vi "test_RS-xxx Read.vi"(8 "error in (no error)":errorcluster, 11 "TestCase in":refnum<class "Instrument Addon Serial Protocols Unit Tests.lvclass">) -> (0 "error out":errorcluster, 3 "TestCase out":refnum<class "Instrument Addon Serial Protocols Unit Tests.lvclass">)   [LabVIEW 2023, in "Instrument Addon Serial Protocols Unit Tests.lvclass"]
uses:
  Instrument Addon Serial Protocols Unit Tests.lvclass
  Instrument Addon Serial Protocols Unit Tests.lvclass/Instrument Addon Serial Protocols Unit Tests.ctl
  <vilib>/addons/_JKI Toolkits/VI Tester/TestCase.llb/TestCase.lvclass
  Listener/Listener.lvclass
  Listener/ListenerClassControls/Operation.ctl
  <vilib>/platform/TimedLoop/XDataNode/XDataNode.xnode
  <vilib>/Platform/TimedLoop/XDataNode/nitl_modes.ctl
  <vilib>/Platform/TimedLoop/XDataNode/XDNodeRunTimeDep.lvlib
  <vilib>/Platform/TimedLoop/XDataNode/wakeup.ctl
  <vilib>/Platform/TimedLoop/XDataNode/timing_clust.ctl
  RS-xxx/RS-xxx.lvclass
  Protocol Parent/Methods/Read Parameter.ctl
  Protocol Parent/Protocol Parent.lvclass
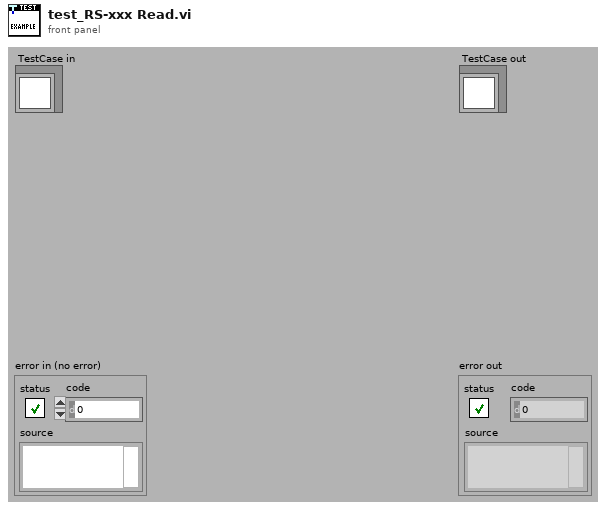
[diagram p1: front panel]
types:
  T1 = typedef "Protocols.lvlib/Protocol Parent.lvclass/Read Parameter.ctl" = cluster{"Wait Type":enum16{"Byte Count", "Wait sec"}, "Wait Value":dbl}
  T2 = typedef "Listener.lvclass/Operation.ctl" = enum16{"Read", "Write"}
  T3 = typedef "XDNodeRunTimeDep.lvlib/timing_clust.ctl" = cluster{"Expected End [f-1]":u64, "Actual End [f-1]":u64, "Finished Late? [f-1]":bool, "Expected End [i-1]":u64, "Actual End [i-1]":u64, "Finished Late? [i-1]":bool, "Expected Start [i]":u64, "Actual Start [i]":u64, "Expected Start [f]":u64, "Actual Start [f]":u64, "Source Name":string, "Structure Name":string, "Period":i64, "Deadline":i64, "Offset":i64, "Start":i64, "Priority":i32, "Timeout":i32, "Mode":T4, "Wakeup Reason":T5, "Error":errorcluster, "Source Type":string, "Secondary Source Type":string, "Global End Time":u64, "Global Start Time":u64, "Frame Duration":u64, "Iteration Duration":u64, "Assigned CPU":i32, "I/O Scan Engine Mode":u32}
  T4 = typedef "XDNodeRunTimeDep.lvlib/nitl_modes.ctl" = enum32{"No Change", "Process missed periods, maintain original phase", "Discard missed periods, maintain original phase", "Process missed periods, ignore original phase", "Discard missed periods, ignore original phase"}
  T5 = typedef "XDNodeRunTimeDep.lvlib/wakeup.ctl" = enum32{"Normal", "Aborted", "Asynchronous wakeup", "Timing source error", "Timed loop error", "Timeout"}
  T6 = typedef "Listener.lvclass/RS-xxx Data Structure.ctl" = cluster{"Virtual COM Port Settings 1":cluster{"Port":string, "Baud Rate":u32, "Data Bits":u16, "Parity":enum16{"None", "Odd", "Even", "Mark", "Space"}, "Stop Bits":u16, "Flow Control":u16, "XON":enum16{"NUL", "SOH", "STX", "ETX", "EOT", "ENQ", "ACK", "BEL", "BS", "HT", "LF", "VT", "FF", "CR", "SO", "SI", "DLE", "DC1", "DC2", "DC3", "DC4", "NAK", "SYN", "ETB", "CAN", "EM", "SUB", "ESC", "FS", "GS", "RS", "US", "SP", "!", "\"", "#", "$", "%", "&", "'", "(", ")", "*", "+", ",", "- (-)", ".", "/", "0", "1", "2", "3", "4", "5", "6", "7", "8", "9", ":", ";", "<", "=", ">", "?", "@", "A", "B", "C", "D", "E", "F", "G", "H", "I", "J", "K", "L", "M", "N", "O", "P", "Q", "R", "S", "T", "U", "V", "W", "X", "Y", "Z", "[", "\\", "]", "^", "_", "`", "a", "b", "c", "d", "e", "f", "g", "h", "i", "j", "k", "l", "m", "n", "o", "p", "q", "r", "s", "t", "u", "v", "w", "x", "y", "z", "{", "|", "}", "~"}, "XOFF":enum16{"NUL", "SOH", "STX", "ETX", "EOT", "ENQ", "ACK", "BEL", "BS", "HT", "LF", "VT", "FF", "CR", "SO", "SI", "DLE", "DC1", "DC2", "DC3", "DC4", "NAK", "SYN", "ETB", "CAN", "EM", "SUB", "ESC", "FS", "GS", "RS", "US", "SP", "!", "\"", "#", "$", "%", "&", "'", "(", ")", "*", "+", ",", "- (-)", ".", "/", "0", "1", "2", "3", "4", "5", "6", "7", "8", "9", ":", ";", "<", "=", ">", "?", "@", "A", "B", "C", "D", "E", "F", "G", "H", "I", "J", "K", "L", "M", "N", "O", "P", "Q", "R", "S", "T", "U", "V", "W", "X", "Y", "Z", "[", "\\", "]", "^", "_", "`", "a", "b", "c", "d", "e", "f", "g", "h", "i", "j", "k", "l", "m", "n", "o", "p", "q", "r", "s", "t", "u", "v", "w", "x", "y", "z", "{", "|", "}", "~"}, "End Read on Termination Character":bool, "End Write on Termination Character":bool, "Termination Character":u8}, "Virtual COM Port Settings 2":cluster{"Port":string, "Baud Rate":u32, "Data Bits":u16, "Parity":enum16{"None", "Odd", "Even", "Mark", "Space"}, "Stop Bits":u16, "Flow Control":u16, "XON":enum16{"NUL", "SOH", "STX", "ETX", "EOT", "ENQ", "ACK", "BEL", "BS", "HT", "LF", "VT", "FF", "CR", "SO", "SI", "DLE", "DC1", "DC2", "DC3", "DC4", "NAK", "SYN", "ETB", "CAN", "EM", "SUB", "ESC", "FS", "GS", "RS", "US", "SP", "!", "\"", "#", "$", "%", "&", "'", "(", ")", "*", "+", ",", "- (-)", ".", "/", "0", "1", "2", "3", "4", "5", "6", "7", "8", "9", ":", ";", "<", "=", ">", "?", "@", "A", "B", "C", "D", "E", "F", "G", "H", "I", "J", "K", "L", "M", "N", "O", "P", "Q", "R", "S", "T", "U", "V", "W", "X", "Y", "Z", "[", "\\", "]", "^", "_", "`", "a", "b", "c", "d", "e", "f", "g", "h", "i", "j", "k", "l", "m", "n", "o", "p", "q", "r", "s", "t", "u", "v", "w", "x", "y", "z", "{", "|", "}", "~"}, "XOFF":enum16{"NUL", "SOH", "STX", "ETX", "EOT", "ENQ", "ACK", "BEL", "BS", "HT", "LF", "VT", "FF", "CR", "SO", "SI", "DLE", "DC1", "DC2", "DC3", "DC4", "NAK", "SYN", "ETB", "CAN", "EM", "SUB", "ESC", "FS", "GS", "RS", "US", "SP", "!", "\"", "#", "$", "%", "&", "'", "(", ")", "*", "+", ",", "- (-)", ".", "/", "0", "1", "2", "3", "4", "5", "6", "7", "8", "9", ":", ";", "<", "=", ">", "?", "@", "A", "B", "C", "D", "E", "F", "G", "H", "I", "J", "K", "L", "M", "N", "O", "P", "Q", "R", "S", "T", "U", "V", "W", "X", "Y", "Z", "[", "\\", "]", "^", "_", "`", "a", "b", "c", "d", "e", "f", "g", "h", "i", "j", "k", "l", "m", "n", "o", "p", "q", "r", "s", "t", "u", "v", "w", "x", "y", "z", "{", "|", "}", "~"}, "End Read on Termination Character":bool, "End Write on Termination Character":bool, "Termination Character":u8}, "Data":string, "Data Length":u32}
  T7 = cluster{"Port":string, "Baud Rate":u32, "Data Bits":u16, "Parity":enum16{"None", "Odd", "Even", "Mark", "Space"}, "Stop Bits":u16, "Flow Control":u16, "XON":enum16{"NUL", "SOH", "STX", "ETX", "EOT", "ENQ", "ACK", "BEL", "BS", "HT", "LF", "VT", "FF", "CR", "SO", "SI", "DLE", "DC1", "DC2", "DC3", "DC4", "NAK", "SYN", "ETB", "CAN", "EM", "SUB", "ESC", "FS", "GS", "RS", "US", "SP", "!", "\"", "#", "$", "%", "&", "'", "(", ")", "*", "+", ",", "- (-)", ".", "/", "0", "1", "2", "3", "4", "5", "6", "7", "8", "9", ":", ";", "<", "=", ">", "?", "@", "A", "B", "C", "D", "E", "F", "G", "H", "I", "J", "K", "L", "M", "N", "O", "P", "Q", "R", "S", "T", "U", "V", "W", "X", "Y", "Z", "[", "\\", "]", "^", "_", "`", "a", "b", "c", "d", "e", "f", "g", "h", "i", "j", "k", "l", "m", "n", "o", "p", "q", "r", "s", "t", "u", "v", "w", "x", "y", "z", "{", "|", "}", "~"}, "XOFF":enum16{"NUL", "SOH", "STX", "ETX", "EOT", "ENQ", "ACK", "BEL", "BS", "HT", "LF", "VT", "FF", "CR", "SO", "SI", "DLE", "DC1", "DC2", "DC3", "DC4", "NAK", "SYN", "ETB", "CAN", "EM", "SUB", "ESC", "FS", "GS", "RS", "US", "SP", "!", "\"", "#", "$", "%", "&", "'", "(", ")", "*", "+", ",", "- (-)", ".", "/", "0", "1", "2", "3", "4", "5", "6", "7", "8", "9", ":", ";", "<", "=", ">", "?", "@", "A", "B", "C", "D", "E", "F", "G", "H", "I", "J", "K", "L", "M", "N", "O", "P", "Q", "R", "S", "T", "U", "V", "W", "X", "Y", "Z", "[", "\\", "]", "^", "_", "`", "a", "b", "c", "d", "e", "f", "g", "h", "i", "j", "k", "l", "m", "n", "o", "p", "q", "r", "s", "t", "u", "v", "w", "x", "y", "z", "{", "|", "}", "~"}, "End Read on Termination Character":bool, "End Write on Termination Character":bool, "Termination Character":u8}
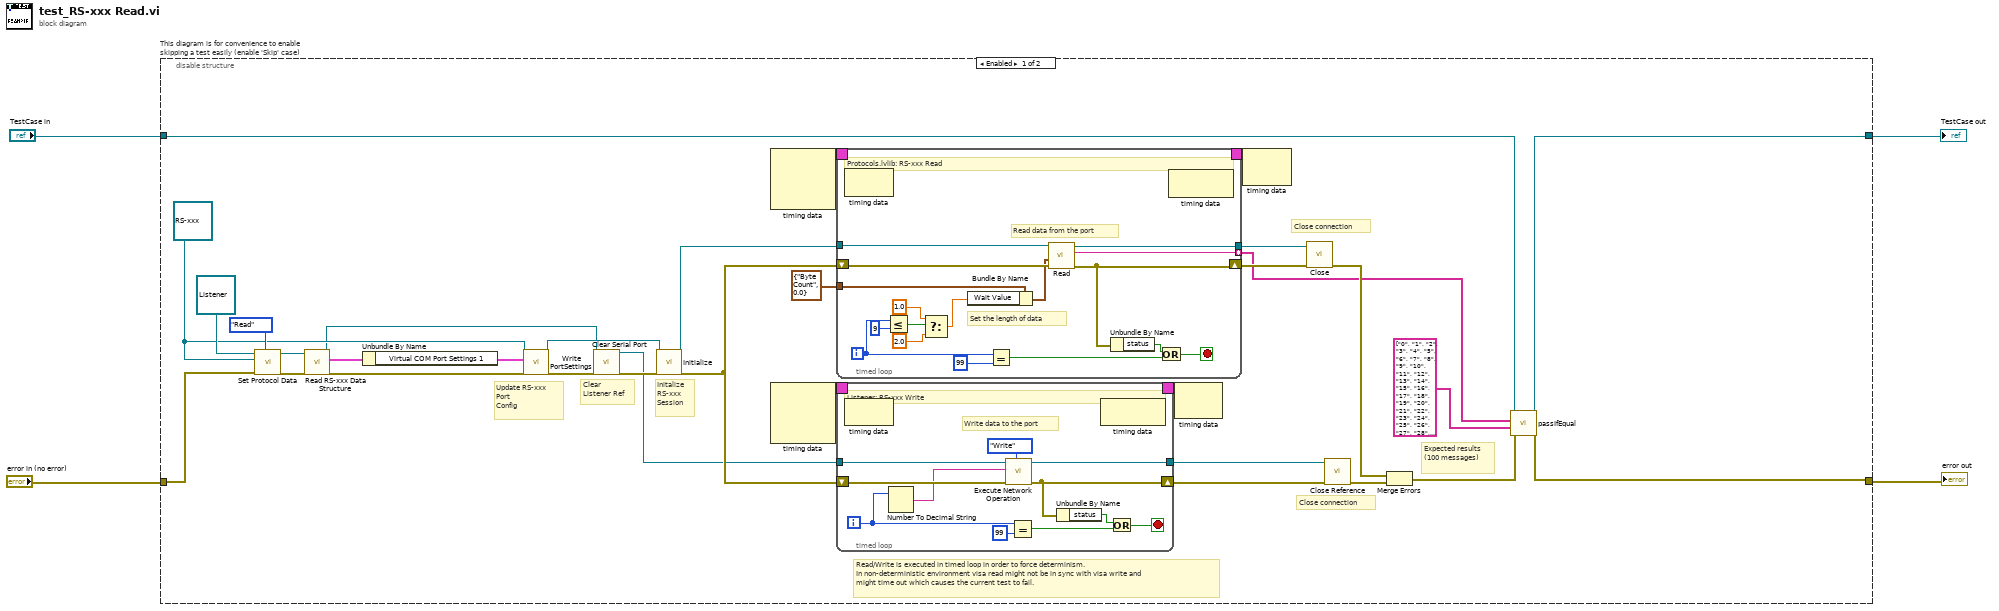
[diagram p0: block diagram]
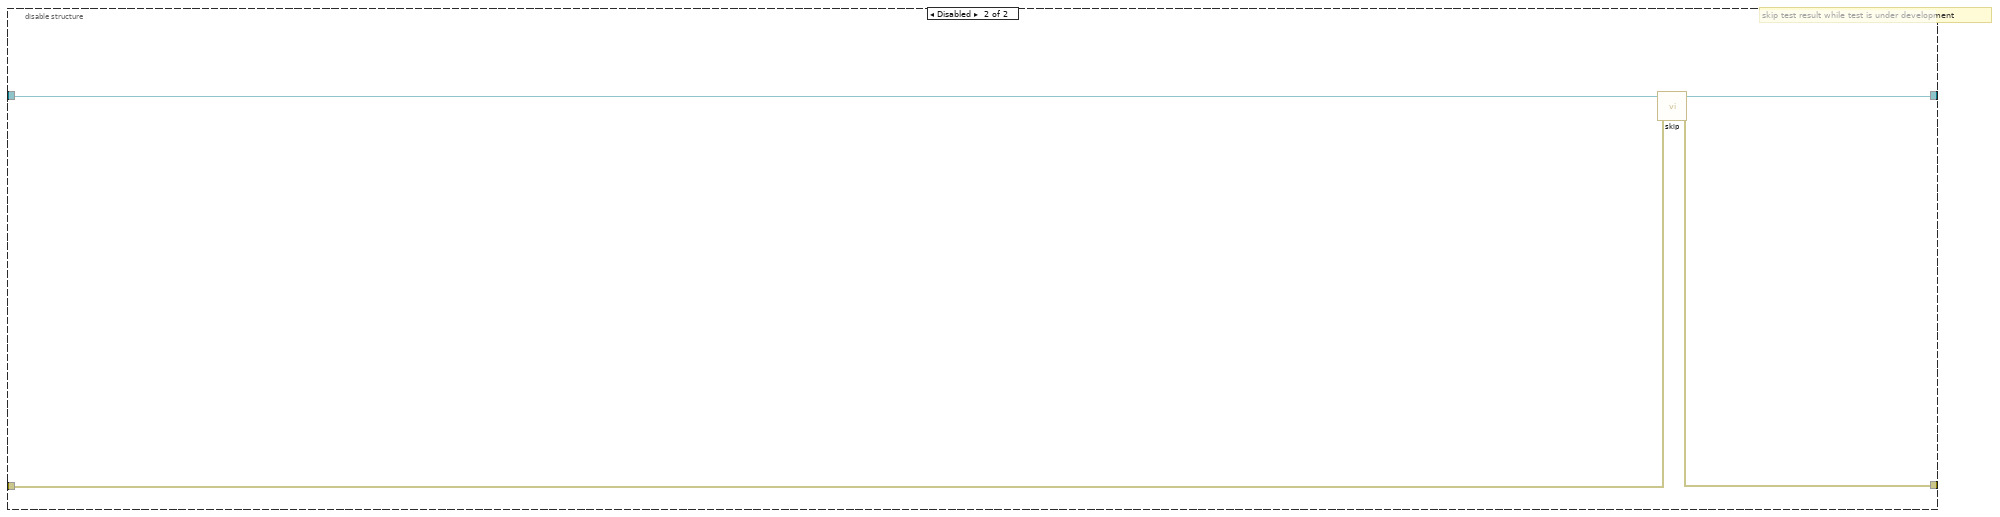
[diagram p2: hidden frame]
diagram:
  n1 = disable-structure "This diagram is for convenience to enable skipping a test easily (enable 'Skip' case)" shown="Enabled" {
    disable-tunnel: "TestCase in" -> [w37 w77]
    disable-tunnel: [w36 w75] -> w2
    disable-tunnel: [w35 w76] -> w4
    disable-tunnel: "error in (no error)" -> [w31 w74]
    frame Enabled {
      w19 = refnum<class "RS-xxx.lvclass"> refnum ("Protocols.lvlib:RS-xxx.lvclass")
      # "Clear \nListener Ref"
      # "Update RS-xxx \nPort \nConfig"
      # "Initalize \nRS-xxx\nSession"
      # "Close connection"
      # "Close connection"
      # "Read/Write is executed in timed loop in order to force determinism.\nIn non-deterministic environment visa read might not be in sync with visa write and\nmight time out which causes the current test to fail."
      # "Expected results\n(100 messages)"
      n2 = call "Set Protocol Data.vi"("Operation"=Operation."Read", "error in (no error)"=w31, "Protocols.lvlib:Protocol Parent.lvclass"=w19, "Listener In.lvclass"=refnum<class "Listener.lvclass"> refnum ("Listener.lvclass")) -> ("error out"=w20:errorcluster, "Listener Out.lvclass"=w21:refnum<class "Listener.lvclass">)  [unwired: 6 in]
      n3 = call-dynamic "Read RS-xxx Data Structure.vi"("error in (no error)"=w20, "Listener in"=w21) -> ("error out"=w16:errorcluster, "RS-xxx Data Structure"=w15:T6, "Listener out"=w9:refnum<class "Listener.lvclass">)  [unwired: 7 in]
      n4 = Unbundle By Name(w15) -> ("Virtual COM Port Settings 1"=w14:T7)
      n5 = call "Write PortSettings.vi"("error in (no error)"=w16, "PortSettings"=w14, "RS232 in"=w19) -> ("error out"=w10:errorcluster, "RS232 out"=w18:refnum<class "RS-xxx.lvclass">)  [unwired: 7 in]
      n6 = call "Clear Serial Port.vi"("error in (no error)"=w10, "Listener In.lvclass"=w9) -> ("error out"=w8:errorcluster, "Listener out"=w5:refnum<class "Listener.lvclass">)  [unwired: 8 in]
      n7 = call-dynamic "Initialize.vi"("error in (no error)"=w8, "RS232 in"=w18) -> ("error out"=w7:errorcluster, "RS232 out"=w17:refnum<class "RS-xxx.lvclass">)  [unwired: 8 in]
      n8 = node-c288() -> (w25:T3)  [unwired: 3 in]
      n9 = node-c288() -> (w23:T3)  [unwired: 3 in]
      n10 = timed-loop {
        shift-right: [w54] -> w28
        shift-left: w7 -> [w66]
        timing: w25 -> [_]
        timing-out: [_] -> w24
        tunnel: w17 -> [w65]
        tunnel: T1 {"Wait Type"=enum."Byte Count", "Wait Value"=0.0} ("Read Parameter") -> [w64]
        tunnel: [w62] -> w12
        tunnel: [w61] -> w11 mode=indexing
        i -> [w60]
        stop <- w67 stop-if-true
        # "Set the length of data"
        # "Read data from the port"
        # "Protocols.lvlib: RS-xxx Read"
        n11 = node-c288() -> ()  [unwired: 1 in, 1 out]
        n12 = Less Or Equal?(x=w60, y=9) -> (x <= y?=w58:bool)
        n13 = Select(t=1.0, s=w58, f=2.0) -> (s? t:f=w55:dbl)
        n14 = Bundle By Name(cluster=w64, "Wait Value"=w55) -> (w63:T1)
        n15 = Equal?(x=w60, y=99) -> (x = y?=w69:bool)
        n16 = call-dynamic "Read.vi"("error in (no error)"=w66, "Variant"=w63, "RS232 in"=w65) -> ("error out"=w54:errorcluster, "String"=w61:string, "RS232 out"=w62:refnum<class "RS-xxx.lvclass">)  [unwired: 6 in]
        n17 = Unbundle By Name(w54) -> ("status"=w53:bool)
        n18 = Or(x=w53, y=w69) -> (x .or. y?=w67:bool)
        n19 = node-c288() -> ()  [unwired: 1 in, 1 out]
      }
      n20 = timed-loop {
        shift-right: [w39] -> w26
        shift-left: w7 -> [w42]
        tunnel: [w44] -> w27
        timing: w23 -> [_]
        timing-out: [_] -> w22
        tunnel: w5 -> [w43]
        i -> [w41]
        stop <- w45 stop-if-true
        # "Write data to the port"
        # "Listener: RS-xxx Write"
        n21 = node-c288() -> ()  [unwired: 1 in, 1 out]
        n22 = Number To Decimal String(number=w41) -> (decimal integer string=w40:string)  [unwired: 1 in]
        n23 = call "Execute Network Operation.vi"("Operation"=Operation."Write", "error in (no error)"=w42, "Message"=w40, "Listener In.lvclass"=w43) -> ("error out"=w39:errorcluster, "Listener Out.lvclass"=w44:refnum<class "Listener.lvclass">)  [unwired: 6 in]
        n24 = Equal?(x=w41, y=99) -> (x = y?=w46:bool)
        n25 = Unbundle By Name(w39) -> ("status"=w38:bool)
        n26 = node-c288() -> ()  [unwired: 1 in, 1 out]
        n27 = Or(x=w38, y=w46) -> (x .or. y?=w45:bool)
      }
      n28 = node-c288(w22) -> ()  [unwired: 1 out]
      n29 = node-c288(w24) -> ()  [unwired: 1 out]
      n30 = call-dynamic "Close.vi"("error in (no error)"=w28, "RS232 in"=w12) -> ("error out"=w30:errorcluster)  [unwired: 8 in, 1 out]
      n31 = call "Close Reference.vi"("error in (no error)"=w26, "Listener In.lvclass"=w27) -> ("error out"=w29:errorcluster)  [unwired: 8 in, 1 out]
      n32 = Merge Errors(w30, w29) -> (w32:errorcluster)
      n33 = call-dynamic "passIfEqual.vi"("error in (no error)"=w32, "y"=string[] ["0", "1", "2", "3", "4", "5", "6", "7", "8", "9", "10", "11", "12", "13", "14", "15", "16", "17", "18", "19", "20", "21", "22", "23", "24", "25", "26", "27", "28", "29", "30", "31", "32", "33", "34", "35", "36", "37", "38", "39", "40", "41", "42", "43", "44", "45", "46", "47", "48", "49", "50", "51", "52", "53", "54", "55", "56", "57", "58", "59", "60", "61", "62", "63", "64", "65", "66", "67", "68", "69", "70", "71", "72", "73", "74", "75", "76", "77", "78", "79", "80", "81", "82", "83", "84", "85", "86", "87", "88", "89", "90", "91", "92", "93", "94", "95", "96", "97", "98", "99"] ("Array"), "x"=w11, "TestCase in"=w37) -> ("error out"=w35:errorcluster, "TestCase out"=w36:refnum<class "Instrument Addon Serial Protocols Unit Tests.lvclass">)  [unwired: 6 in]
    }
    frame Disabled {
      # "skip test result while test is under development"
      n34 = call <vilib>:"skip.vi"("error in (no error)"=w74, "TestCase in"=w77) -> ("error out"=w76:errorcluster, "TestCase out"=w75:refnum<class "Instrument Addon Serial Protocols Unit Tests.lvclass">)  [unwired: 8 in]
    }
  }
  "error out" <- w4
  "TestCase out" <- w2
